vi "HTML Data Global.vi"(0 "HTML refnum":u32, 5 "menu":enum16{"init", "get", "set", "delete"}(ring), 9 "HTML report data in":T1) -> (4 "HTML refnum out":u32, 10 "HTML report data out":T1)   [LabVIEW 2015, in "NI_ReportGenerationCore.lvlib"]
uses:
  <vilib>/Utility/NIReport.llb/NI_ReportGenerationCore.lvlib
  <vilib>/Utility/NIReport.llb/HTML Report Data.ctl
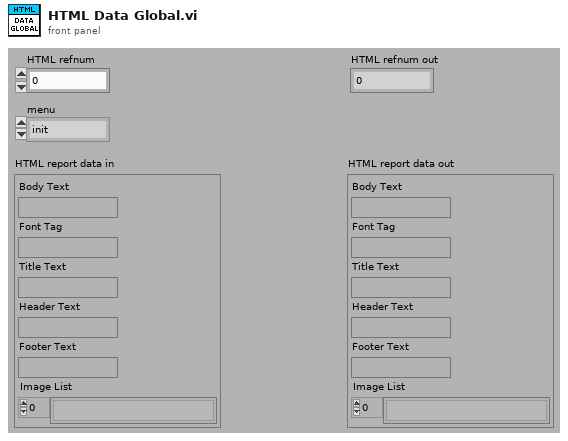
[diagram p1: front panel]
types:
  T1 = typedef "NI_ReportGenerationCore.lvlib/HTML Report Data.ctl" = cluster{"Body Text":string, "Font Tag":string, "Title Text":string, "Header Text":string, "Footer Text":string, "Image List":path[]}
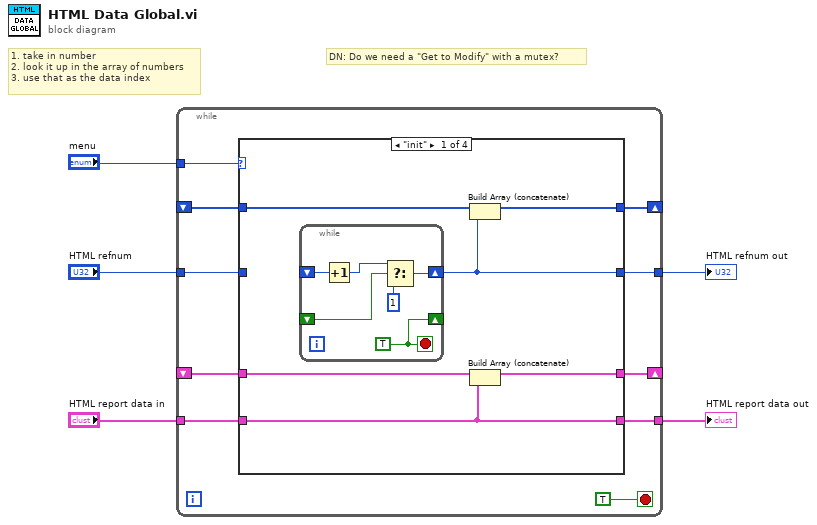
[diagram p0: block diagram]
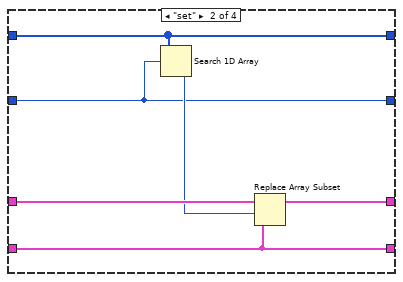
[diagram p2: hidden frame]
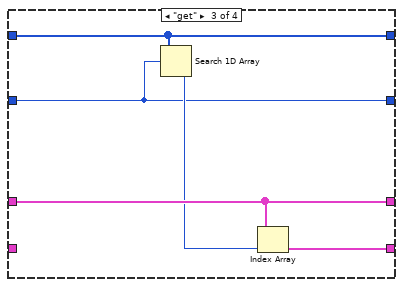
[diagram p3: hidden frame]
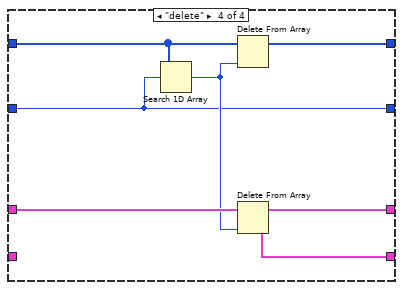
[diagram p4: hidden frame]
diagram:
  # "DN: Do we need a \"Get to Modify\" with a mutex?"
  # "1. take in number\n2. look it up in the array of numbers\n3. use that as the data index"
  n1 = while {
    tunnel: "menu" -> [w15]
    shift-right: [w14] -> _
    shift-left: _ -> [w13]
    tunnel: "HTML refnum" -> [w11]
    shift-right: [w9] -> _
    shift-left: _ -> [w10]
    tunnel: [w8] -> w3
    tunnel: "HTML report data in" -> [w7]
    tunnel: [w6] -> w1
    stop <- TRUE stop-if-true
    n2 = case shown="\"init\"" w15 {
      tunnel: [w21 w31 w37 w42] -> w14
      tunnel: w13 -> [w20 w32 w37 w43]
      tunnel: w11 -> [_ w28 w34 w39]
      tunnel: w10 -> [w19 w33 w35 w45]
      tunnel: [w18 w33 w35 w44] -> w9
      tunnel: [w17 w29 w38 w40] -> w8
      tunnel: w7 -> [w17 w29 _ _]
      tunnel: [w16 w28 w34 w39] -> w6
      frame "init" {
        n3 = while {
          shift-right: [w26] -> w16
          shift-left: _ -> [w27]
          shift-right: [w25] -> _
          shift-left: _ -> [w22]
          stop <- w25 stop-if-true
          w25 = TRUE
          n4 = Increment(x=w27) -> (x+1=w24:u32)
          n5 = Select(t=w24, s=w22, f=u32 1 ("HTML refnum out")) -> (s? t:f=w26:u32)
        }
        n6 = Build Array (concatenate)(w19, w16) -> (w18:u32[])
        n7 = Build Array (concatenate)(w20, w17) -> (w21:T1[])
      }
      frame "set" {
        n8 = Search 1D Array(1D array=w33, element=w28) -> (index of element=w30:i32)  [unwired: 1 out]
        n9 = Replace Array Subset(array=w32, new element=w29, index=w30) -> (w31:T1[])
      }
      frame "get" {
        n10 = Search 1D Array(1D array=w35, element=w34) -> (index of element=w36:i32)  [unwired: 1 out]
        n11 = Index Array(array=w37, index=w36) -> (element=w38:T1)
      }
      frame "delete" {
        n12 = Search 1D Array(1D array=w45, element=w39) -> (index of element=w41:i32)  [unwired: 1 out]
        n13 = Delete From Array(array=w45, index=w41) -> (array with subset deleted=w44:u32[])  [unwired: 1 in, 1 out]
        n14 = Delete From Array(array=w43, index=w41) -> (deleted portion=w40:T1, array with subset deleted=w42:T1[])  [unwired: 1 in]
      }
    }
  }
  "HTML report data out" <- w3
  "HTML refnum out" <- w1
